vi "P5.vi"() -> ()   [LabVIEW 2018]
uses:
  <vilib>/picture/picture.llb/Draw True-Color Pixmap.vi
  <vilib>/vision/NI_Vision_Development_Module.lvlib
  <vilib>/picture/picture.llb/Draw 4-Bit Pixmap.vi
panel:
  out "error out":errorcluster
  in  "stop":bool
  out "2D Picture":picture
  in  "Image Type":T1 items=["Grayscale (U8)", "Grayscale (I16)", "Grayscale (SGL)", "Complex (CSG)", "RGB (U32)", "HSL (U32)", "RGB (U64)", "Grayscale (U16)"]
  in  "error in (no error)":errorcluster
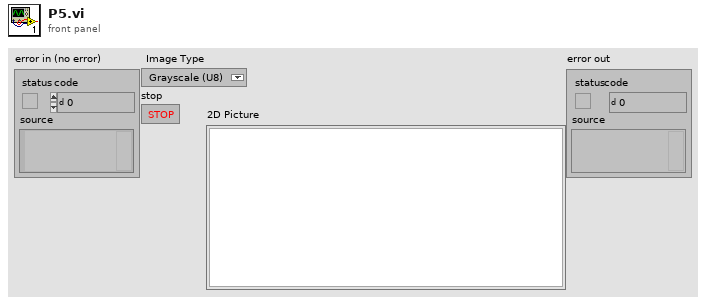
[diagram p1: front panel]
types:
  T1 = typedef "Image Type" = u32
  T2 = typedef "IMAQ Image.ctl" = refnum<image>
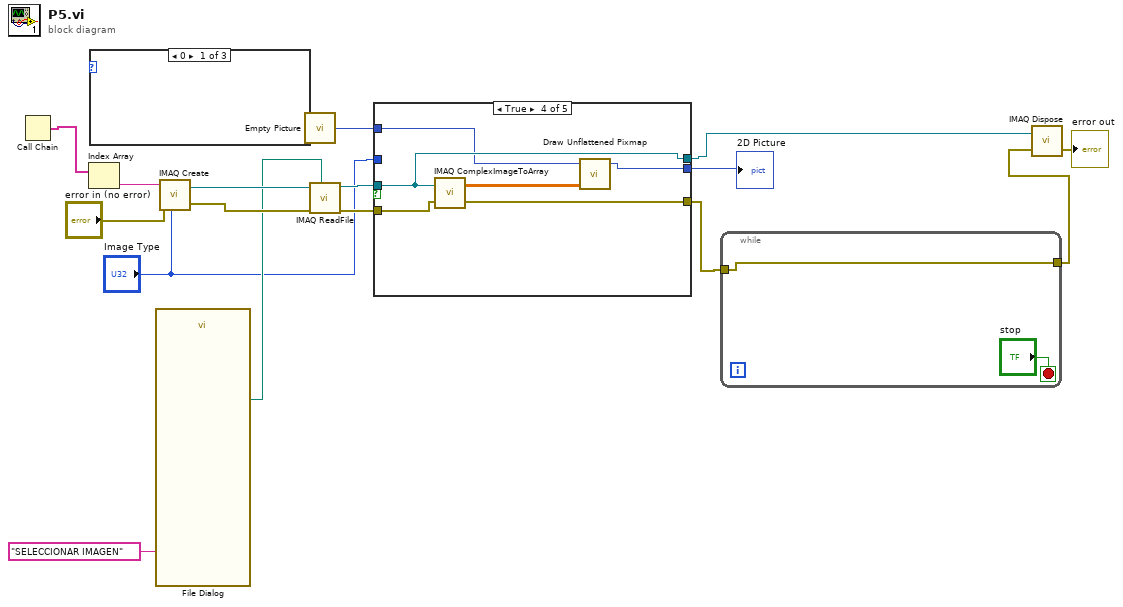
[diagram p0: block diagram]
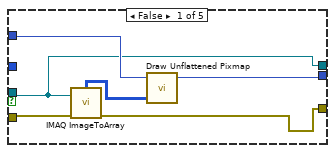
[diagram p4: hidden frame]
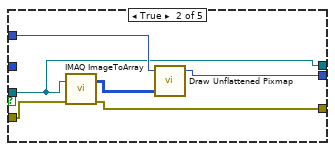
[diagram p5: hidden frame]
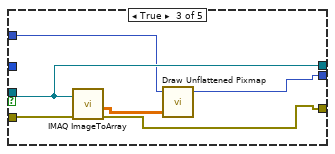
[diagram p6: hidden frame]
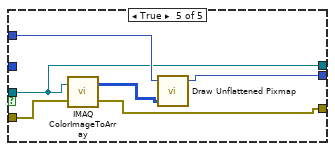
[diagram p7: hidden frame]
diagram:
  n1 = Call Chain() -> (call chain=w16:string[])
  n2 = Index Array(array=w16) -> (element=w15:string)  [unwired: 1 in]
  n3 = case shown="0" {
    selector: _ -> [_ _ _]
    frame 0 {
    }
    frame 1 {
    }
    frame 2 {
    }
  }
  n4 = call "File Dialog"("prompt"="SELECCIONAR IMAGEN") -> ("selected path"=w10:path)  [unwired: 11 in, 3 out]
  n5 = call "IMAQ Create"("Image Name"=w15, "Image Type"="Image Type", "error in (no error)"="error in (no error)") -> ("New Image"=w14:T2, "error out"=w13:errorcluster)  [unwired: 2 in]
  n6 = call "Empty Picture"() -> ("empty picture"=w6:picture)
  n7 = call <userlib>:"IMAQ ReadFile.vi"("File Path"=w10, "error in (no error)"=w13, "Image"=w14) -> ("error out"=w8:errorcluster, "Image Out"=w9:T2)  [unwired: 4 in, 3 out]
  n8 = case shown="\"1\"" {
    selector: _ -> [_ _ _ _ _]
    tunnel: w9 -> [w17 w24 w33 w39 w44]
    tunnel: w8 -> [w22 w28 w34 w40 w46]
    tunnel: "Image Type" -> [_ _ _ _ _]
    tunnel: w6 -> [w21 w27 w32 w38 w45]
    tunnel: [w17 w24 w33 w39 w44] -> w2
    tunnel: [w19 w25 w29 w36 w41] -> w4
    tunnel: [w18 w26 w30 w35 w43] -> w5
    frame False {
      n9 = call "IMAQ ImageToArray"("error in (no error)"=w22, "Image"=w17) -> ("error out"=w19:errorcluster, "Image Pixels (U8)"=w20:u8[][])  [unwired: 2 in, 3 out]
      n10 = call-poly <vilib>:"Draw Unflattened Pixmap.vi"("picture"=w21, "data"=w20) -> ("new picture"=w18:picture)  [unwired: 7 in]
    }
    frame True {
      n11 = call "IMAQ ImageToArray"("error in (no error)"=w28, "Image"=w24) -> ("error out"=w25:errorcluster, "Image Pixels (I16)"=w23:i16[][])  [unwired: 2 in, 3 out]
      n12 = call-poly <vilib>:"Draw Unflattened Pixmap.vi"("picture"=w27, "data (RGB format)"=w23) -> ("new picture"=w26:picture)  [unwired: 7 in]
    }
    frame True {
      n13 = call "IMAQ ImageToArray"("error in (no error)"=w34, "Image"=w33) -> ("Image Pixels (Float)"=w31:sgl[][], "error out"=w29:errorcluster)  [unwired: 2 in, 3 out]
      n14 = call-poly <vilib>:"Draw Unflattened Pixmap.vi"("picture"=w32, "data (RGB format)"=w31) -> ("new picture"=w30:picture)  [unwired: 7 in]
    }
    frame True {
      n15 = call "IMAQ ComplexImageToArray"("Image"=w39, "error in (no error)"=w40) -> ("Image Pixels (Complex)"=w37:csg[][], "error out"=w36:errorcluster)  [unwired: 3 in]
      n16 = call-poly <vilib>:"Draw Unflattened Pixmap.vi"("picture"=w38, "data (RGB format)"=w37) -> ("new picture"=w35:picture)  [unwired: 7 in]
    }
    frame True {
      n17 = call "IMAQ ColorImageToArray"("Image"=w44, "error in (no error)"=w46) -> ("Image Pixels (U32)"=w42:u32[][], "error out"=w41:errorcluster)  [unwired: 2 in, 1 out]
      n18 = call-poly <vilib>:"Draw Unflattened Pixmap.vi"("picture"=w45, "data (RGB format)"=w42) -> ("new picture"=w43:picture)  [unwired: 7 in]
    }
  }
  "2D Picture" <- w5
  n19 = while {
    tunnel: w4 -> [w47]
    tunnel: [w47] -> w3
    stop <- "stop" stop-if-true
  }
  n20 = call "IMAQ Dispose"("Image"=w2, "error in (no error)"=w3) -> ("error out"=→"error out":errorcluster)  [unwired: 4 in]
